vi "Working example.vi"() -> ()   [LabVIEW 2025]
panel:
  out "Waveform Graph":waveform(dbl)[](graph)
  out "error out":errorcluster
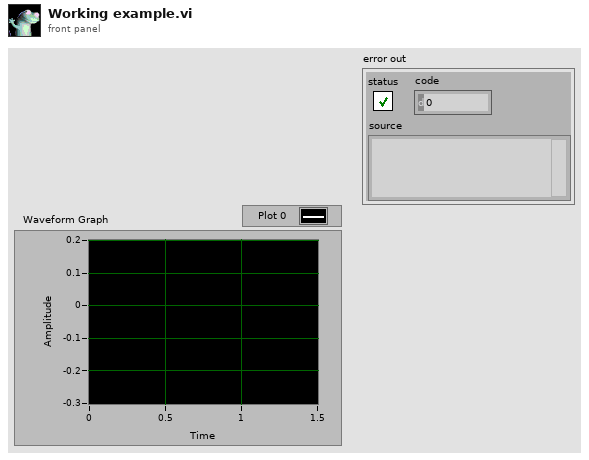
[diagram p1: front panel]
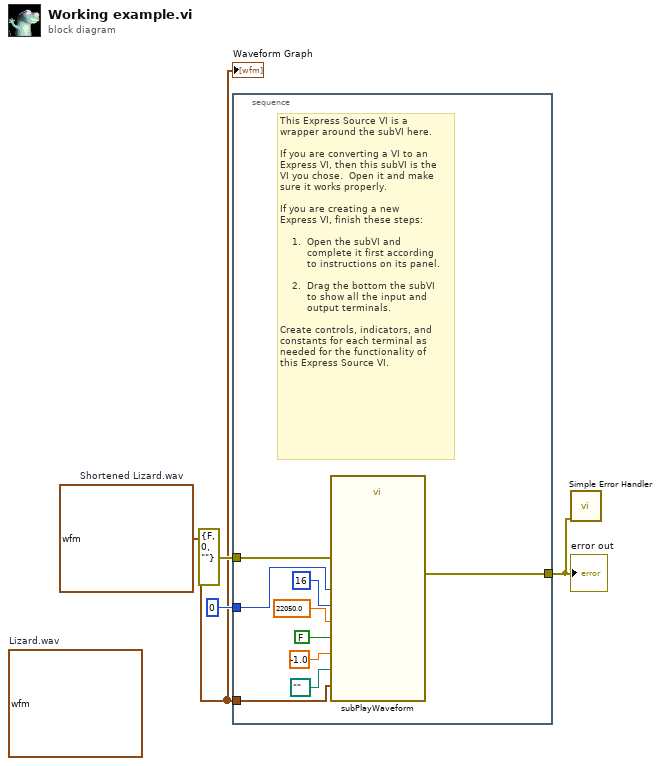
[diagram p0: block diagram]
diagram:
  w1 = waveform(dbl)[] [{"t0"=timestamp(0 s since 1904-01-01), "dt"=2.0833333333333333e-05, "Y"=array[22560 elements]}, {"t0"=timestamp(0 s since 1904-01-01), "dt"=2.0833333333333333e-05, "Y"=array[22560 elements]}]  # Shortened Lizard.wav
  (unwired) waveform(dbl)[] [{"t0"=timestamp(0 s since 1904-01-01), "dt"=2.0833333333333333e-05, "Y"=array[57600 elements]}, {"t0"=timestamp(0 s since 1904-01-01), "dt"=2.0833333333333333e-05, "Y"=array[57600 elements]}]  # Lizard.wav
  n1 = stacked-sequence {
    tunnel: u32 0 ("Device") -> [w11]
    tunnel: w1 -> [w9]
    tunnel: errorcluster {"status"=FALSE, "code"=0, "source"=""} ("error in") -> [w5]
    tunnel: [w12] -> w4
    frame #0 {
      # "This Express Source VI is a \nwrapper around the subVI here.  \n\nIf you are converting a VI to an\nExpress VI, then this subVI is the\nVI you chose.  Open it and make \nsure it works properly.\n\nIf you are creating a new \nExpress VI, finish these steps:\n\n    1.  Open the subVI and \n         complete it first according \n         to instructions on its panel.\n\n    2.  Drag the bottom the subVI \n         to show all the input and \n         output terminals.\n\nCreate controls, indicators, and \nconstants for each terminal as \nneeded for the functionality of \nthis Express Source VI."
      n2 = call <vilib>:"subPlayWaveform.vi"("Device"=w11, "Resolution (bits)"=16, "Sample rate (Hz)"=22050.0, "Use rate"=FALSE, "Path"=path "", "error in (no error)"=w5, "Data"=w9, "Timeout (sec)"=-1.0) -> ("error out"=w12:errorcluster)  [unwired: 11 in]
    }
  }
  "error out" <- w4
  n3 = call <vilib>:"Simple Error Handler.vi"("error in (no error)"=w4) -> ()  [unwired: 4 in, 5 out]
  "Waveform Graph" <- w1
